vi "Write Cabin.vi"(8 "error in (no error)":errorcluster, 10 "Cabin":bool, 11 "Change Inlet MSG in":refnum<class "Change Inlet MSG.lvclass">) -> (0 "error out":errorcluster, 3 "Change Inlet MSG out":refnum<class "Change Inlet MSG.lvclass">)   [LabVIEW 2014]
uses:
  Change Inlet MSG.lvclass
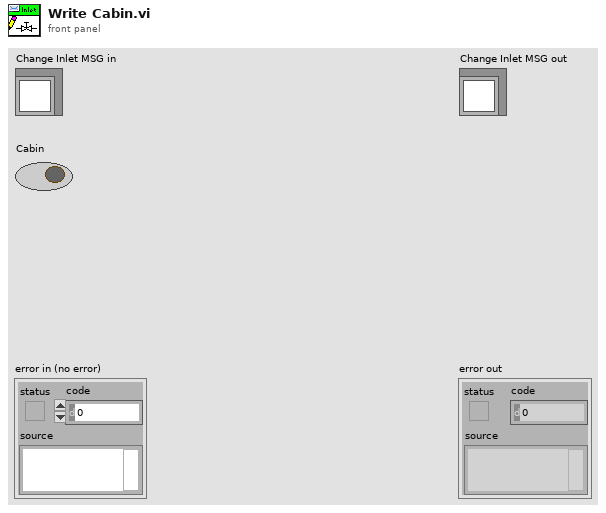
[diagram p1: front panel]
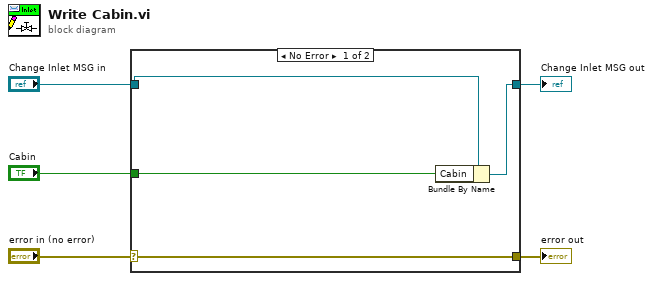
[diagram p0: block diagram]
diagram:
  n1 = case shown="No Error" "error in (no error)" {
    selector: "error in (no error)" -> [w9 w10]
    tunnel: [w9 w10] -> w4
    tunnel: [w7 w11] -> w2
    tunnel: "Change Inlet MSG in" -> [w8 w11]
    tunnel: "Cabin" -> [w6 _]
    frame No Error {
      n2 = Bundle By Name(cluster=w8, "Cabin"=w6) -> (w7:refnum<class "Change Inlet MSG.lvclass">)
    }
    frame Error {
    }
  }
  "error out" <- w4
  "Change Inlet MSG out" <- w2
